vi "Configure Control Mode.vi"(8 "error in (no error)":errorcluster, 9 "control mode":u8(ring) items=["setpoint = BUS setpoint", "setpoint = analog input", "setpoint = master output(FLOW-BUS) * slave factor(FLOW-BUS)", "close valve", "controller idle", "testmode enable", "tuningmode enable", "setpoint = 100%", "purge valve", "calibration mode enable", "setpoint = master output(analog in) * slave factor(FLOW-BUS)", "setpoint = keyboard OR FLOW-BUS setpoint", "setpoint = 0%", "setpoint = master output(FLOW-BUS) * slave factor(analog in)", "(FPP) range select mode", "(FPP) manual start sensor select, automatic end sensor", "(FPP) automatic start sensor select, manual end sensor", "(FPP) automatic start and end sensor", "setpoint = RS232 setpoint", "RS232 broadcast mode", "valve stearing", "analog valve stearing", "valve safe state"], 10 "node":u8, 11 "ProPar in":refnum<class "PL Bronkhorst ProPar.lvclass">) -> (0 "error out":errorcluster, 3 "ProPar out":refnum<class "PL Bronkhorst ProPar.lvclass">)   [LabVIEW 2015, in "PL Bronkhorst ProPar.lvclass"]
doc: "Configures control mode of the specified <b>node</b>."
uses:
  PL Bronkhorst ProPar.lvclass
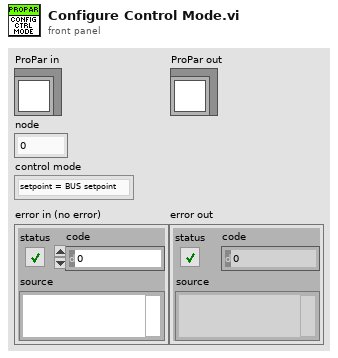
[diagram p1: front panel]
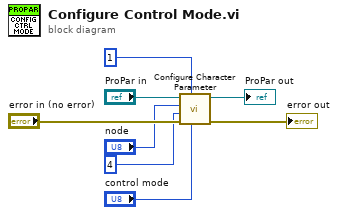
[diagram p0: block diagram]
diagram:
  n1 = call "Configure Character Parameter.vi"("value"="control mode", "process number"=u8 1, "error in (no error)"="error in (no error)", "parameter number"=u8 4 ("process number"), "node"="node", "ProPar in"="ProPar in") -> ("error out"=→"error out":errorcluster, "ProPar out"=→"ProPar out":refnum<class "PL Bronkhorst ProPar.lvclass">)  [unwired: 4 in]
